vi "RenderRobotPose.vi"(0 "Robot X (in)":dbl, 1 "Robot Width (in)":dbl=30.0 format="%#_13g", 2 "Robot Length (in)":dbl=30.0 format="%#_13g", 3 "Buffer Time (min)":dbl=5.0 format="%#_13g", 5 "Robot Y (in)":dbl, 7 "Targeting Information":dbl[](array[numeric])=[0.0, 0.0, 0.0, 0.0], 9 "Robot Heading (deg)":dbl, 11 "Planned Path":T2, 12 "Robot Enabled":bool, 13 "Seen_Game_Pieces":T1(array[cluster]), 14 "Reset":bool) -> (6 "Robot Pose":cluster{dbl[], dbl[]}[](graph))   [LabVIEW 2020]
doc: "This VI takes the robot pose information as input and renders a plot to display it. At this time, only square robot dimensions are supported."
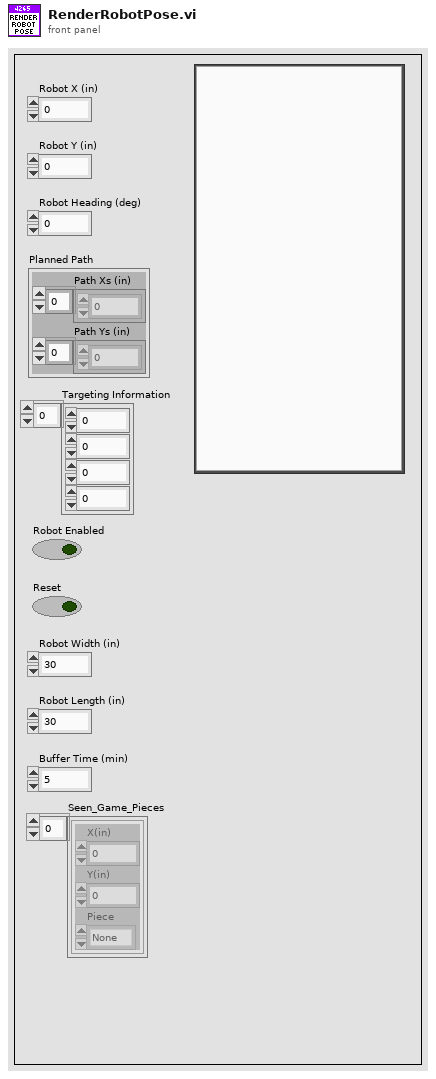
[diagram p1: front panel]
types:
  T1 = cluster{"X(in)":dbl, "Y(in)":dbl, "Piece":enum16{"None", "Cube", "Cone"}}[]
  T2 = cluster{"Path Xs (in)":dbl[], "Path Ys (in)":dbl[]}
  T3 = cluster{"Path Xs (in)":dbl[], "Path Ys (in)":dbl[]}[]
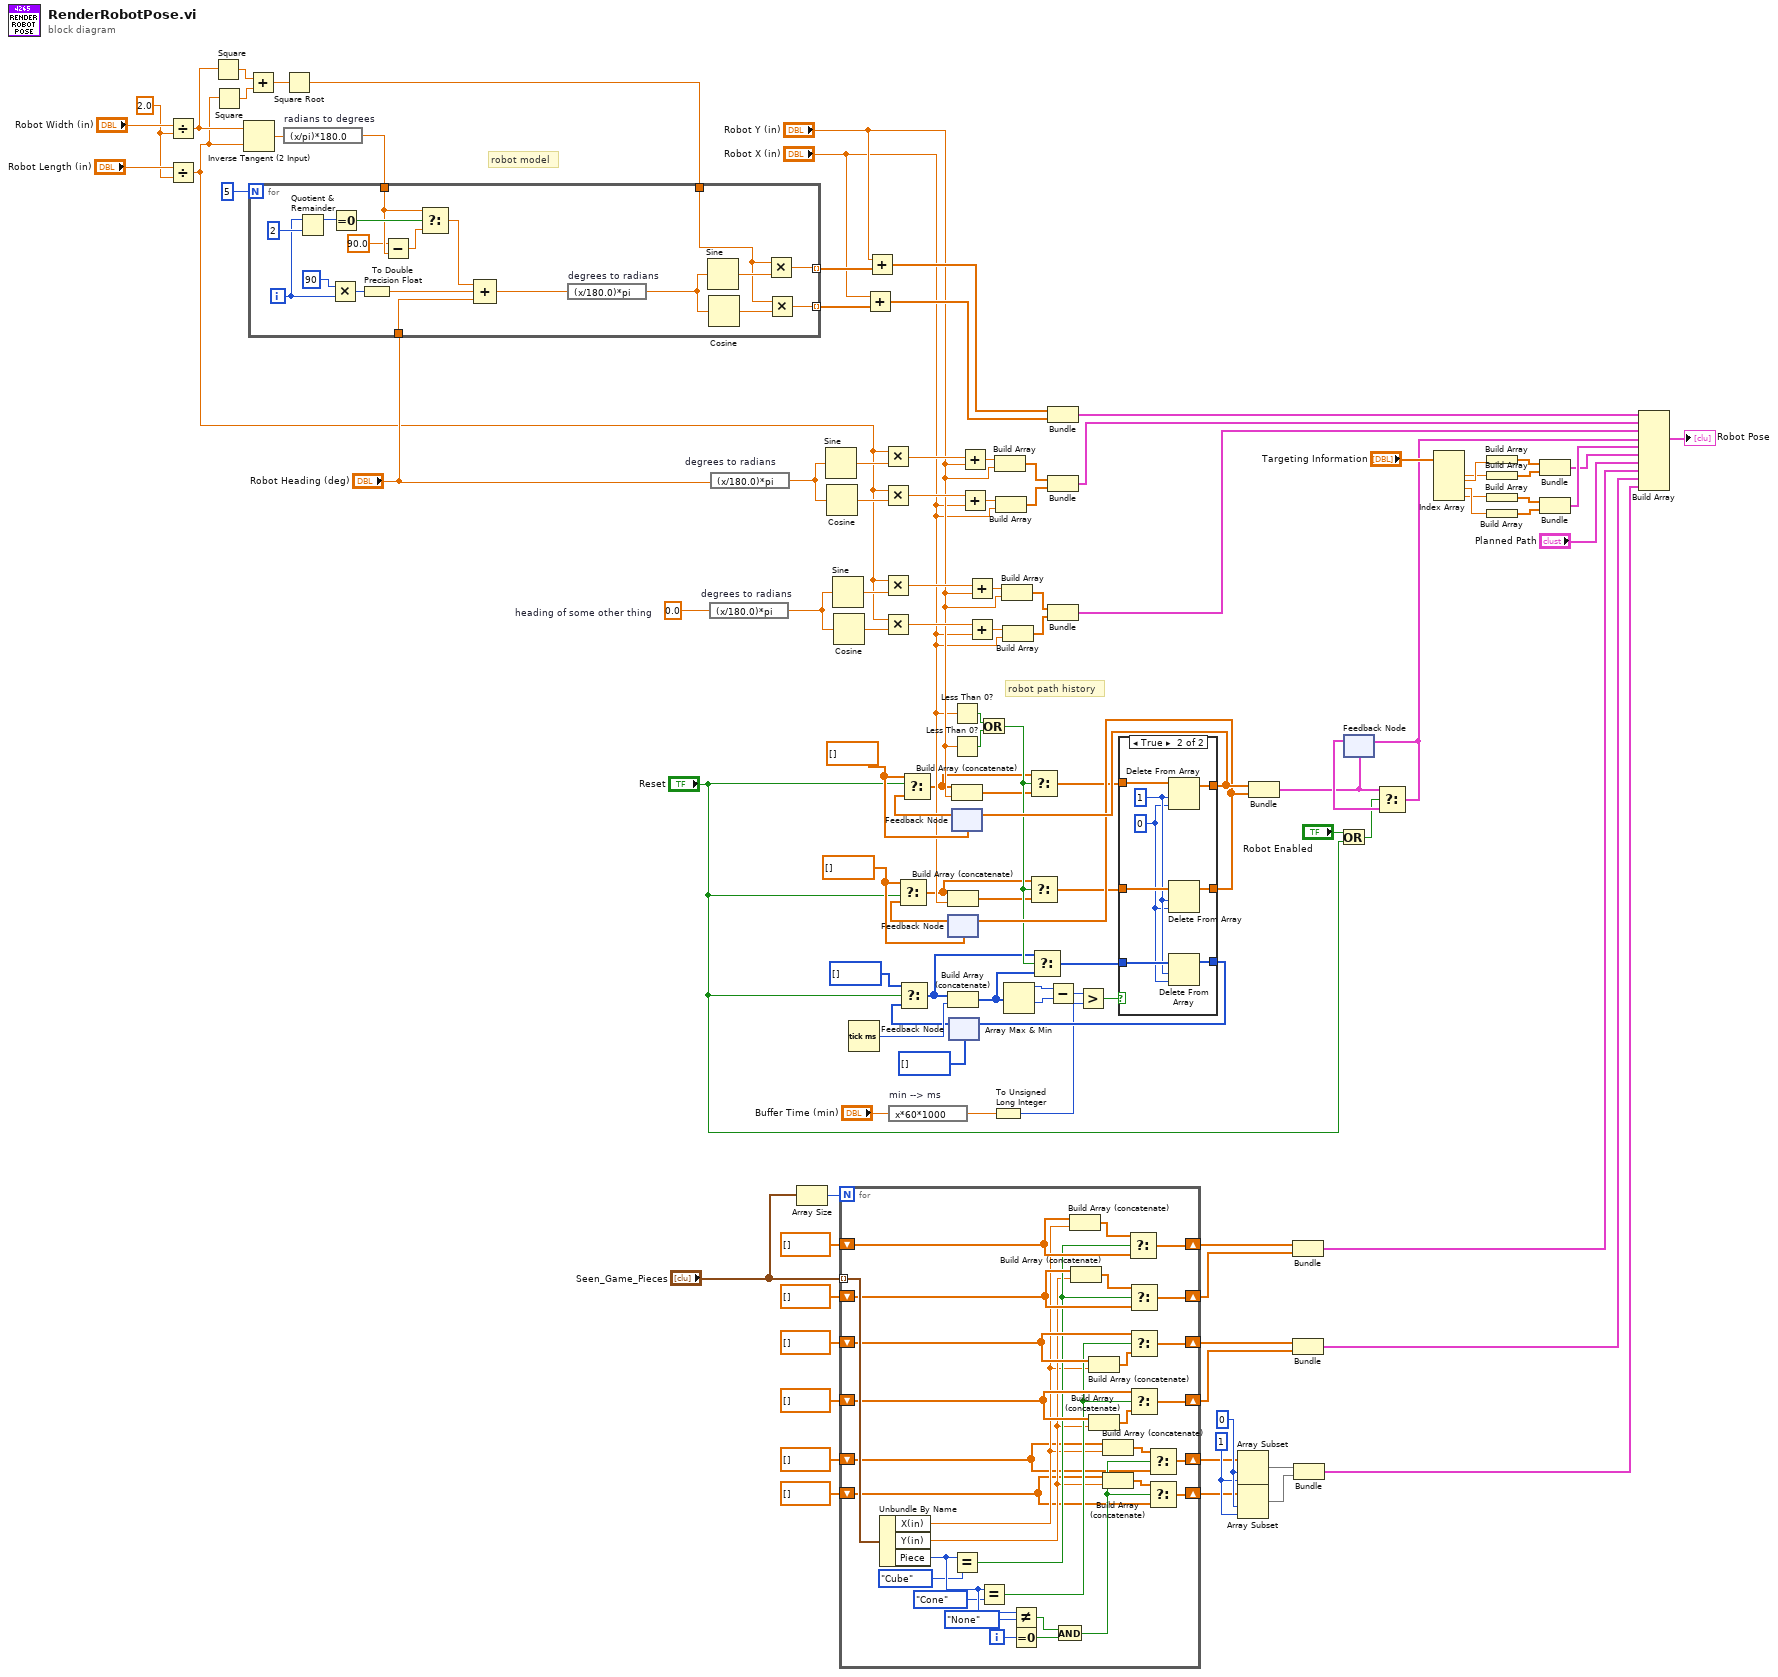
[diagram p0: block diagram]
diagram:
  w9 = 1 ("length")
  w19 = 0 ("index")
  w29 = 0.0  # heading of some other thing
  w47 = 2.0
  w66 = dbl[] [] ("t")
  w65 = dbl[] [] ("t")
  # "robot model"
  # "robot path history"
  n1 = Divide(x="Robot Width (in)", y=w47) -> (x/y=w44:dbl)
  n2 = Divide(x="Robot Length (in)", y=w47) -> (x/y=w43:dbl)
  n3 = Square(x=w44) -> (x^2=w41:dbl)
  n4 = Square(x=w43) -> (x^2=w42:dbl)
  n5 = Inverse Tangent (2 Input)(1:w43, 2:w44) -> (0:w46:dbl)
  n6 = Add(x=w41, y=w42) -> (x+y=w40:dbl)
  n7 = Square Root(x=w40) -> (sqrt(x)=w39:dbl)
  n8 = expression code="(x/pi)*180.0" "radians to degrees"(w46) -> (w45:dbl)
  n9 = for {
    N: 5 -> [_]
    tunnel: [w127] -> w110 mode=indexing
    tunnel: [w126] -> w109 mode=indexing
    tunnel: "Robot Heading (deg)" -> [w121]
    tunnel: w45 -> [w117]
    tunnel: w39 -> [w112]
    i -> [w113]
    n10 = Quotient & Remainder(x=w113, y=2) -> (x-y*floor(x/y)=w119:i32)  [unwired: 1 out]
    n11 = Multiply(x=90, y=w113) -> (x*y=w124:i32)
    n12 = Equal To 0?(x=w119) -> (x = 0?=w118:bool)
    n13 = To Double Precision Float(number=w124) -> (double precision float=w123:dbl)
    n14 = Subtract(x=90.0, y=w117) -> (x-y=w116:dbl)
    n15 = Select(t=w117, s=w118, f=w116) -> (s? t:f=w114:dbl)
    n16 = Compound Arithmetic op=ADD(w114, w123, w121) -> (w122:dbl)
    n17 = expression code="(x/180.0)*pi" "degrees to radians"(w122) -> (w129:dbl)
    n18 = Sine(x=w129) -> (sin(x)=w128:dbl)
    n19 = Cosine(x=w129) -> (cos(x)=w130:dbl)
    n20 = Multiply(x=w112, y=w128) -> (x*y=w126:dbl)
    n21 = Multiply(x=w112, y=w130) -> (x*y=w127:dbl)
  }
  n22 = expression code="(x/180.0)*pi" "degrees to radians"(w29) -> (w88:dbl)
  n23 = expression code="(x/180.0)*pi" "degrees to radians"("Robot Heading (deg)") -> (w79:dbl)
  n24 = Array Size(array="Seen_Game_Pieces") -> (size(s)=w21:i32)
  n25 = Sine(x=w79) -> (sin(x)=w78:dbl)
  n26 = Cosine(x=w79) -> (cos(x)=w77:dbl)
  n27 = Sine(x=w88) -> (sin(x)=w87:dbl)
  n28 = Cosine(x=w88) -> (cos(x)=w86:dbl)
  n29 = for {
    N: w21 -> [_]
    tunnel: "Seen_Game_Pieces" -> [w161] mode=indexing
    shift-right: [w159] -> w13
    shift-left: dbl[] [] -> [w158]
    shift-right: [w156] -> w12
    shift-left: dbl[] [] -> [w155]
    shift-right: [w153] -> w8
    shift-left: dbl[] [] -> [w152]
    shift-right: [w154] -> w7
    shift-left: dbl[] [] -> [w150]
    shift-right: [w142] -> w4
    shift-left: dbl[] [] -> [w136]
    shift-right: [w141] -> w3
    shift-left: dbl[] [] -> [w137]
    i -> [w146]
    n30 = Unbundle By Name(w161) -> ("X(in)"=w138:dbl, "Y(in)"=w139:dbl, "Piece"=w144:enum16{"None", "Cube", "Cone"})
    n31 = Equal?(x=w144, y=enum16{"None", "Cube", "Cone"}."Cube") -> (x = y?=w148:bool)
    n32 = Equal?(x=w144, y=enum16{"None", "Cube", "Cone"}."Cone") -> (x = y?=w147:bool)
    n33 = Not Equal?(x=w144, y=enum16{"None", "Cube", "Cone"}."None") -> (x != y?=w143:bool)
    n34 = Equal To 0?(x=w146) -> (x = 0?=w145:bool)
    n35 = And(x=w143, y=w145) -> (x .and. y?=w140:bool)
    n36 = Build Array (concatenate)(w158, w138) -> (w160:dbl[])
    n37 = Build Array (concatenate)(w155, w139) -> (w157:dbl[])
    n38 = Build Array (concatenate)(w152, w138) -> (w151:dbl[])
    n39 = Build Array (concatenate)(w150, w139) -> (w149:dbl[])
    n40 = Build Array (concatenate)(w136, w138) -> (w132:dbl[])
    n41 = Build Array (concatenate)(w137, w139) -> (w131:dbl[])
    n42 = Select(t=w160, s=w148, f=w158) -> (s? t:f=w159:dbl[])
    n43 = Select(t=w157, s=w148, f=w155) -> (s? t:f=w156:dbl[])
    n44 = Select(t=w152, s=w147, f=w151) -> (s? t:f=w153:dbl[])
    n45 = Select(t=w150, s=w147, f=w149) -> (s? t:f=w154:dbl[])
    n46 = Select(t=w132, s=w140, f=w136) -> (s? t:f=w142:dbl[])
    n47 = Select(t=w131, s=w140, f=w137) -> (s? t:f=w141:dbl[])
  }
  n48 = Tick Count (ms)() -> (millisecond timer value=w93:u32)
  n49 = Add(x="Robot X (in)", y=w110) -> (x+y=w107:dbl[])
  n50 = Add(x="Robot Y (in)", y=w109) -> (x+y=w106:dbl[])
  n51 = Multiply(x=w43, y=w78) -> (x*y=w76:dbl)
  n52 = Multiply(x=w43, y=w77) -> (x*y=w75:dbl)
  n53 = Multiply(x=w43, y=w87) -> (x*y=w85:dbl)
  n54 = Multiply(x=w43, y=w86) -> (x*y=w84:dbl)
  n55 = expression code="x*60*1000" "min --> ms"("Buffer Time (min)") -> (w98:dbl)
  n56 = feedback #1(w65) -> (w89:dbl[])
  n57 = Select(t=w65, s="Reset", f=w89) -> (s? t:f=w54:dbl[])
  n58 = Build Array (concatenate)(w54, "Robot X (in)") -> (w55:dbl[])
  n59 = feedback #2(u32[] []) -> (w91:u32[])
  n60 = Select(t=u32[] [], s="Reset", f=w91) -> (s? t:f=w59:u32[])
  n61 = Build Array (concatenate)(w59, w93) -> (w58:u32[])
  n62 = Less Than 0?(x="Robot X (in)") -> (x < 0?=w62:bool)
  n63 = Less Than 0?(x="Robot Y (in)") -> (x < 0?=w63:bool)
  n64 = feedback #3(w66) -> (w92:dbl[])
  n65 = Select(t=w66, s="Reset", f=w92) -> (s? t:f=w56:dbl[])
  n66 = Build Array (concatenate)(w56, "Robot Y (in)") -> (w57:dbl[])
  n67 = Add(x=w76, y="Robot Y (in)") -> (x+y=w74:dbl)
  n68 = Add(x=w75, y="Robot X (in)") -> (x+y=w73:dbl)
  n69 = Add(x=w85, y="Robot Y (in)") -> (x+y=w83:dbl)
  n70 = Add(x=w84, y="Robot X (in)") -> (x+y=w82:dbl)
  n71 = Or(x=w62, y=w63) -> (x .or. y?=w61:bool)
  n72 = To Unsigned Long Integer(number=w98) -> (unsigned 32bit integer=w99:u32)
  n73 = Build Array(w74, "Robot Y (in)") -> (w72:dbl[])
  n74 = Build Array(w73, "Robot X (in)") -> (w71:dbl[])
  n75 = Build Array(w83, "Robot Y (in)") -> (w81:dbl[])
  n76 = Build Array(w82, "Robot X (in)") -> (w80:dbl[])
  n77 = Array Max & Min(array=w58) -> (max value=w95:u32, min value=w96:u32)  [unwired: 2 out]
  n78 = Select(t=w56, s=w61, f=w57) -> (s? t:f=w68:dbl[])
  n79 = Select(t=w54, s=w61, f=w55) -> (s? t:f=w67:dbl[])
  n80 = Select(t=w59, s=w61, f=w58) -> (s? t:f=w60:u32[])
  n81 = Bundle(w106, w107) -> (w23:cluster{dbl[], dbl[]})  [unwired: 1 in]
  n82 = Bundle(w72, w71) -> (w26:cluster{dbl[], dbl[]})  [unwired: 1 in]
  n83 = Bundle(w81, w80) -> (w27:cluster{dbl[], dbl[]})  [unwired: 1 in]
  n84 = Subtract(x=w95, y=w96) -> (x-y=w97:u32)
  n85 = Greater?(x=w97, y=w99) -> (0:w101:bool)
  n86 = case shown="True" w101 {
    tunnel: w60 -> [w162 w170]
    tunnel: w67 -> [w163 w171]
    tunnel: w68 -> [w164 w172]
    tunnel: [w164 w167] -> w104
    tunnel: [w163 w166] -> w103
    tunnel: [w162 w165] -> w102
    frame False {
    }
    frame True {
      w168 = 0 ("index")
      w169 = 1 ("length")
      n87 = Delete From Array(array=w172, length=w169, index=w168) -> (array with subset deleted=w167:dbl[])  [unwired: 1 out]
      n88 = Delete From Array(array=w171, length=w169, index=w168) -> (array with subset deleted=w166:dbl[])  [unwired: 1 out]
      n89 = Delete From Array(array=w170, length=w169, index=w168) -> (array with subset deleted=w165:u32[])  [unwired: 1 out]
    }
  }
  n90 = feedback-in #1(w103) -> ()
  n91 = feedback-in #2(w102) -> ()
  n92 = feedback-in #3(w104) -> ()
  n93 = Array Subset(array=w4, index=w19, length=w9) -> (w18:dbl[])
  n94 = Array Subset(array=w3, index=w19, length=w9) -> (w17:dbl[])
  n95 = Bundle("t"=w104, "t"=w103) -> (w70:cluster{"t":dbl[], "t":dbl[]})  [unwired: 1 in]
  n96 = Bundle(w13, w12) -> (w11:cluster{dbl[], dbl[]})  [unwired: 1 in]
  n97 = Bundle(w8, w7) -> (w10:cluster{dbl[], dbl[]})  [unwired: 1 in]
  n98 = Bundle(w18, w17) -> (w16:cluster{dbl[], dbl[]})  [unwired: 1 in]
  n99 = Or(x="Robot Enabled", y="Reset") -> (x .or. y?=w51:bool)
  n100 = feedback #4(w70) -> (w105:cluster{"t":dbl[], "t":dbl[]})
  n101 = Select(t=w70, s=w51, f=w105) -> (s? t:f=w25:cluster{"t":dbl[], "t":dbl[]})
  n102 = feedback-in #4(w25) -> ()
  n103 = Index Array(array="Targeting Information") -> (element #1=w32:dbl, element #2=w33:dbl, element #3=w31:dbl, element #4=w30:dbl)  [unwired: 4 in]
  n104 = Build Array(w33) -> (w38:dbl[])
  n105 = Build Array(w32) -> (w37:dbl[])
  n106 = Build Array(w30) -> (w36:dbl[])
  n107 = Build Array(w31) -> (w35:dbl[])
  n108 = Bundle(w38, w37) -> (w22:cluster{dbl[], dbl[]})  [unwired: 1 in]
  n109 = Bundle(w36, w35) -> (w24:cluster{dbl[], dbl[]})  [unwired: 1 in]
  n110 = Build Array(w23, w26, w27, w25, w24, w22, "Planned Path", w11, w10, w16) -> (→"Robot Pose":T3)
